vi "PDO link.vi"(4 "Map":cluster{"Multiplexor":T1, "nBits":u8}[](array[cluster])=[{"Multiplexor"={"Index"=24832, "Sub-Index"=1}, "nBits"=16}] {"Multiplexor"."Sub-Index" format="%.0x"; "Multiplexor"."Index" format="%04x"}, 5 "Wait?":bool, 6 "error in (no error)":errorcluster, 7 "Indices":cluster{"Communication":u32, "Mapping":u32}={"Communication"=6144, "Mapping"=6656} {"Mapping" format="%x"; "Communication" format="%x"}, 8 "Cob ID":u32, 9 "CANopen in":refnum<class "CANopen.lvclass">) -> (0 "error out":errorcluster, 3 "CANopen out":refnum<class "CANopen.lvclass">)   [LabVIEW 2026, in "canopen_.lvlib" / "CANopen.lvclass"]
doc: "Links a PDO COB-ID to a specific map of OD items."
uses:
  CANopen.lvclass
  CANopen.lvclass/CANopen.ctl
  Multiplexor.ctl
  CANopen Master.lvlib
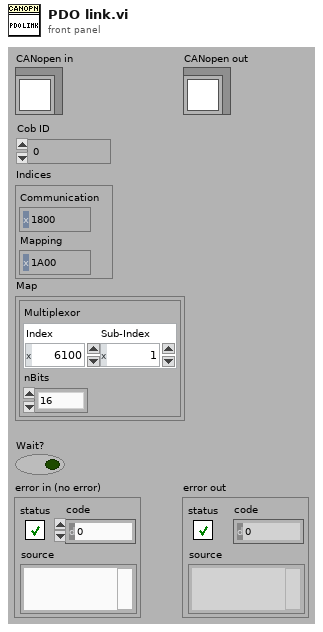
[diagram p1: front panel]
types:
  T1 = typedef "CANopen Master.lvlib/Multiplexor.ctl" = cluster{"Index":u16, "Sub-Index":i16}
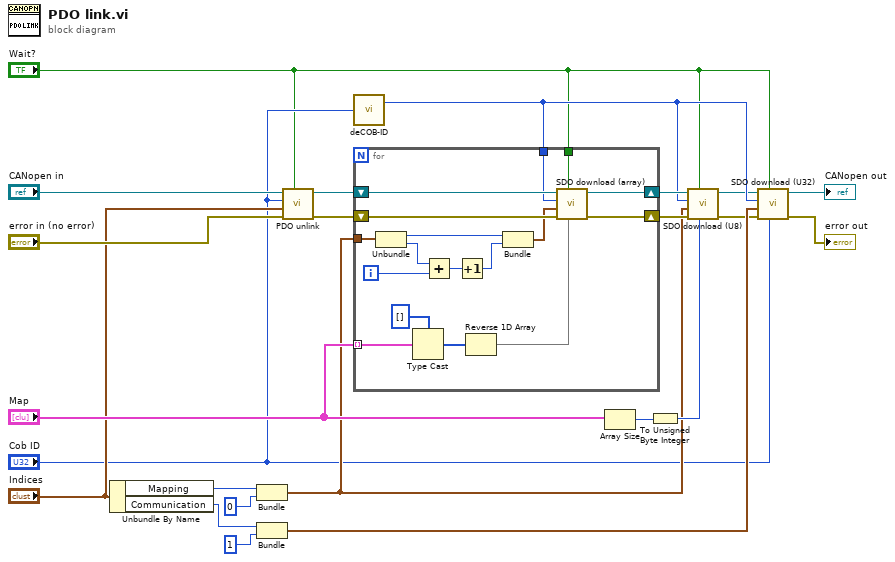
[diagram p0: block diagram]
diagram:
  n1 = Unbundle By Name("Indices") -> ("Mapping"=w14:u32, "Communication"=w7:u32)
  n2 = Bundle("Mapping"=w14, "Sub-index"=u8 0) -> (w15:cluster{"Mapping":u32, "Sub-index":u8})  [unwired: 1 out]
  n3 = Bundle("Communication"=w7, "Sub-index"=u8 1) -> (w21:cluster{"Communication":u32, "Sub-index":u8})  [unwired: 1 out]
  n4 = call "PDO unlink.vi"("Wait?"="Wait?", "error in (no error)"="error in (no error)", "Indices"="Indices", "Cob ID"="Cob ID", "CANopen in"="CANopen in") -> ("error out"=w10:errorcluster, "CANopen out"=w9:refnum<class "CANopen.lvclass">)  [unwired: 2 out]
  n5 = call "deCOB-ID.vi"("Cob ID"="Cob ID") -> ("Node ID"=w13:u8)  [unwired: 1 out]
  n6 = for {
    tunnel: "Map" -> [w36] mode=indexing
    tunnel: w13 -> [w38]
    tunnel: w15 -> [w32]
    shift-right: [w25] -> w17
    shift-left: w10 -> [w39]
    shift-right: [w26] -> w18
    shift-left: w9 -> [w40]
    tunnel: "Wait?" -> [w24]
    i -> [w29]
    n7 = Unbundle(w32) -> ("Mapping"=w31:u32, "Sub-index"=w30:u8)
    n8 = Type Cast(type=u8[] [] ("appended array"), x=w36) -> (*(type *) &x=w34:u8[])
    n9 = Add(x=w30, y=w29) -> (x+y=w28:u8)
    n10 = Increment(x=w28) -> (x+1=w27:u8)
    n11 = Reverse 1D Array(array=w34) -> (reversed array=w33:u8[])
    n12 = Bundle("Mapping"=w31, w27) -> (w37:cluster{"Mapping":u32, u8})  [unwired: 1 out]
    n13 = call "SDO download (array).vi"("Value"=w33, "Wait?"=w24, "error in"=w39, "Multiplexor"=w37, "Node ID"=w38, "CANopen in"=w40) -> ("error out"=w25:errorcluster, "CANopen out"=w26:refnum<class "CANopen.lvclass">)  [unwired: 4 in]
  }
  n14 = Array Size(array="Map") -> (size(s)=w20:i32)
  n15 = To Unsigned Byte Integer(number=w20) -> (unsigned 8bit integer=w19:u8)
  n16 = call "SDO download (U8).vi"("Value"=w19, "Wait?"="Wait?", "error in (no error)"=w17, "Multiplexor"=w15, "Node ID"=w13, "CANopen in"=w18) -> ("error out"=w5:errorcluster, "CANopen out"=w6:refnum<class "CANopen.lvclass">)  [unwired: 4 in]
  n17 = call "SDO download (U32).vi"("Value"="Cob ID", "Wait?"="Wait?", "error in (no error)"=w5, "Multiplexor"=w21, "Node ID"=w13, "CANopen in"=w6) -> ("error out"=→"error out":errorcluster, "CANopen out"=→"CANopen out":refnum<class "CANopen.lvclass">)  [unwired: 4 in]
